vi "20-sub-multiplier.vi"(8 "N2":u8[](array[numeric]), 11 "N1":u8[](array[numeric])) -> (3 "N1*N2":u8[](array[numeric]))   [LabVIEW 2021]
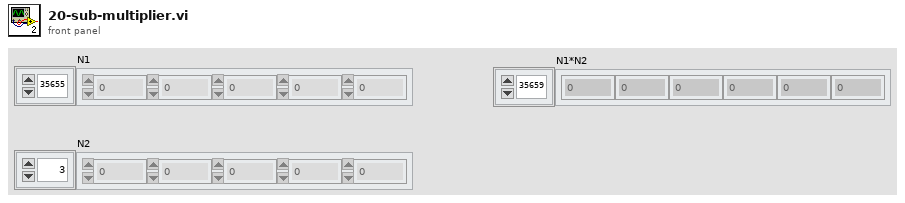
[diagram p1: front panel]
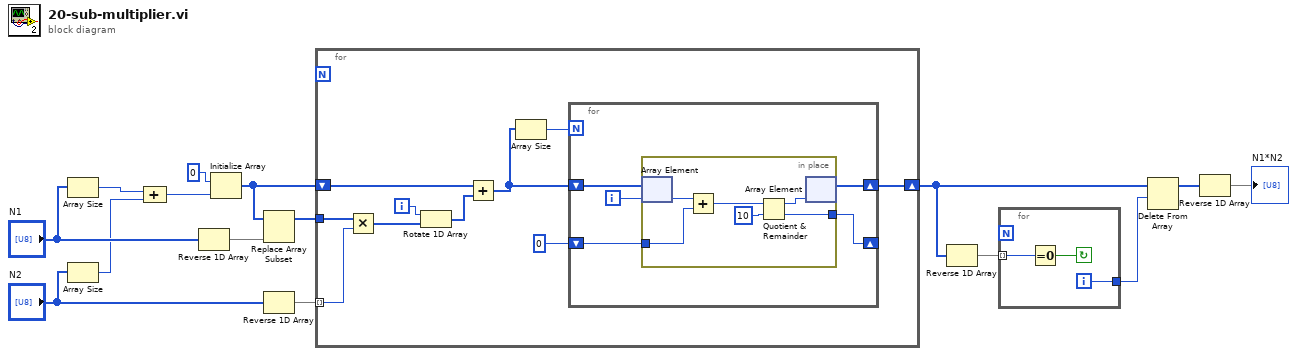
[diagram p0: block diagram]
diagram:
  n1 = Array Size(array="N1") -> (size(s)=w11:i32)
  n2 = Array Size(array="N2") -> (size(s)=w10:i32)
  n3 = Compound Arithmetic op=ADD(w11, w10) -> (w9:i32)
  n4 = Reverse 1D Array(array="N1") -> (reversed array=w6:u8[])
  n5 = Initialize Array(u8 0, w9) -> (w7:u8[])
  n6 = Replace Array Subset(array=w7, new element=w6) -> (w5:u8[])  [unwired: 1 in]
  n7 = Reverse 1D Array(array="N2") -> (reversed array=w14:u8[])
  n8 = for {
    tunnel: w14 -> [w25] mode=indexing
    shift-right: [w19] -> w15
    shift-left: w7 -> [w20]
    tunnel: w5 -> [w21]
    i -> [w17]
    n9 = Multiply(x=w21, y=w25) -> (x*y=w23:u8[])
    n10 = Rotate 1D Array(1:w23, 2:w17) -> (0:w18:u8[])
    n11 = Add(x=w20, y=w18) -> (x+y=w16:u8[])
    n12 = Array Size(array=w16) -> (size(s)=w22:i32)
    n13 = for {
      N: w22 -> [_]
      shift-right: [w29] -> w19
      shift-left: w16 -> [w30]
      shift-right: [w26] -> _
      shift-left: u8 0 -> [w27]
      i -> [w28]
      n14 = in-place {
        in-place-border: w27 -> [w32]
        in-place-border: [w31] -> w26
        n15 = in-place-array #1(w30, w28) -> (w36:u8)
        n16 = Add(x=w36, y=w32) -> (x+y=w33:u8)
        n17 = Quotient & Remainder(x=w33, y=u8 10) -> (x-y*floor(x/y)=w34:u8, floor(x/y)=w31:u8)
        n18 = in-place-array #1(w34) -> (w29:u8[])  [unwired: 1 out]
      }
    }
  }
  n19 = Reverse 1D Array(array=w15) -> (reversed array=w4:u8[])
  n20 = for {
    tunnel: w4 -> [w39] mode=indexing
    tunnel: [w37] -> w3
    i -> [w37]
    stop <- w38 continue-if-true
    n21 = Equal To 0?(x=w39) -> (x = 0?=w38:bool)
  }
  n22 = Delete From Array(array=w15, length=w3) -> (array with subset deleted=w2:u8[])  [unwired: 1 in, 1 out]
  n23 = Reverse 1D Array(array=w2) -> (reversed array=→"N1*N2":u8[])
